vi "E2E Tag Exchange Module.vi"   [LabVIEW 2015]
uses:
  <vilib>/Platform/browser.llb/Open URL in Default Browser (string).vi
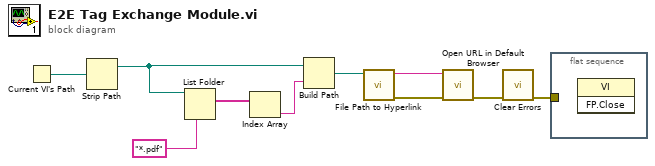
[diagram p0: block diagram]
diagram:
  n1 = Current VI's Path() -> (path=w10:path)
  n2 = Strip Path(path=w10) -> (stripped path=w6:path)  [unwired: 1 out]
  n3 = List Folder(path=w6, pattern="*.pdf") -> (filenames=w8:string[])  [unwired: 1 in, 4 out]
  n4 = Index Array(array=w8) -> (element=w7:string)  [unwired: 1 in]
  n5 = Build Path(base path=w6, name or relative path=w7) -> (appended path=w5:path)
  n6 = call "File Path to Hyperlink.vi"("File Path"=w5) -> ("error out"=w2:errorcluster, "Hyperlink"=w4:string)  [unwired: 9 in]
  n7 = call-poly <vilib>:"Open URL in Default Browser.vi"("error in (no error)"=w2, "URL"=w4) -> ("error out"=w3:errorcluster)  [unwired: 4 in, 1 out]
  n8 = call <vilib>:"Clear Errors.vi"("error in (no error)"=w3) -> ("error out"=w1:errorcluster)  [unwired: 5 in, 1 out]
  n9 = flat-sequence {
    tunnel: w1 -> [_]
    frame #0 {
      n10 = invoke class="VI" method="FP.Close"() -> ()  [unwired: 3 in, 3 out]
    }
  }
